vi "Read.vi"(8 "error in (no error)":errorcluster, 11 "Devantech SRF05 in":refnum<class "Devantech SRF05.lvclass">) -> (0 "error out":errorcluster, 1 "Timeout":bool, 2 "Distance (cm)":dbl, 3 "Devantech SRF05 out":refnum<class "Devantech SRF05.lvclass">)   [LabVIEW 2019, in "Devantech SRF05.lvclass"]
doc: "Reads distance from sensor."
uses:
  Devantech SRF05.lvclass
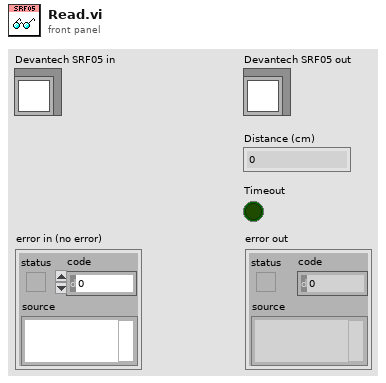
[diagram p1: front panel]
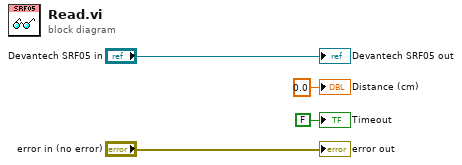
[diagram p0: block diagram]
diagram:
  "Distance (cm)" <- 0.0 ("Distance (cm)")
  "Timeout" <- FALSE ("Timeout")
  "Devantech SRF05 out" <- "Devantech SRF05 in"
  "error out" <- "error in (no error)"
